vi "Do Core.vi"(8 "error in (no error)":errorcluster, 9 "Actor in":refnum<class "Actor.lvclass">, 11 "Reply Message":refnum<class "Write Settings to Ini File.lvclass">) -> (0 "error out":errorcluster, 1 "Actor out":refnum<class "Actor.lvclass">, 2 "Reply":variant)   [LabVIEW 2014, in "Camera Actor.lvlib" / "Write Settings to Ini File.lvclass"]
doc: "(<B>Filename</B>: Actor Framework.lvlib:Reply Msg.lvclass:Do Core.vi)\n\nDefines what an actor does when it receives <B>Reply Message</B>. This method also defines the <B>Reply</B> that is returned to the actor that sent <B>Reply Message</B>.\n\nBy default, this method does nothing, and <B>Reply</B> is the ancestor Message class. A child class must override this method to define behavior and specify a child of the Message class to return in the <B>Reply</B> output."
uses:
  Write Settings to Ini File.lvclass
  <vilib>/ActorFramework/Actor/Actor.lvclass
  Camera Actor/Camera Actor.lvclass
  Write Settings to Ini File.lvclass/Write Settings to Ini File.ctl
  <vilib>/ActorFramework/Reply Msg/Reply Msg.lvclass
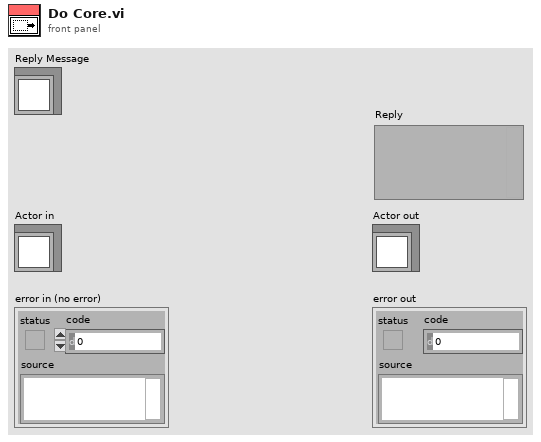
[diagram p1: front panel]
types:
  T1 = typedef "NI_LVConfig.lvlib/Config Data RefNum.ctl" = refnum<k1>
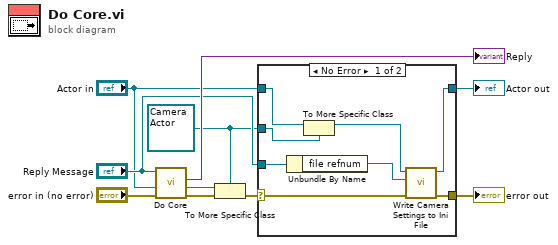
[diagram p0: block diagram]
diagram:
  w1 = refnum<class "Camera Actor.lvclass"> refnum ("IMAQdx Actor.lvlib:IMAQdx Actor.lvclass")
  n1 = call-parent "Do Core.vi"("error in (no error)"="error in (no error)", "Actor in"="Actor in", "Reply Message"="Reply Message") -> ("error out"=w7:errorcluster, "Actor out"=w8:refnum<class "Actor.lvclass">, "Reply"=→"Reply":variant)  [unwired: 6 in]
  n2 = To More Specific Class(target class=w1, reference=w8, error in=w7) -> (error out=w5:errorcluster)  [unwired: 1 out]
  n3 = case shown="No Error" w5 {
    selector: w5 -> [w17 w19]
    tunnel: [w18 w20] -> w6
    tunnel: [w16 w19] -> w4
    tunnel: "Reply Message" -> [w15 _]
    tunnel: "Actor in" -> [w13 w20]
    tunnel: w1 -> [w12 _]
    frame No Error {
      n4 = Unbundle By Name(w15) -> ("file refnum"=w14:T1)
      n5 = To More Specific Class(target class=w12, reference=w13) -> (specific class reference=w11:refnum<class "Camera Actor.lvclass">)  [unwired: 1 in, 1 out]
      n6 = call-dynamic "Write Camera Settings to Ini File.vi"("error in (no error)"=w17, "refnum in"=w14, "Camera in"=w11) -> ("error out"=w16:errorcluster, "Camera out"=w18:refnum<class "Camera Actor.lvclass">)  [unwired: 6 in, 1 out]
    }
    frame Error {
    }
  }
  "error out" <- w4
  "Actor out" <- w6
